vi "checkBeginPassPlay.vi"(8 "error in (no error)":errorcluster, 10 "Game":refnum<class "Game.lvclass">, 11 "PassPlay in":refnum<class "PassPlay.lvclass">) -> (0 "error out":errorcluster, 2 "Boolean":bool, 3 "PassPlay out":refnum<class "PassPlay.lvclass">)   [LabVIEW 2023, in "PassPlay.lvclass"]
uses:
  PassPlay.lvclass
  Game_class/Game.lvclass
  Utilities_class/Utilities.lvclass
  Referee_class/command_interpreted.ctl
  Game_class/Game.lvclass/Game.ctl
  Referee_class/Referee.lvclass/Referee.ctl
  Game_class/Read Referee.vi
  Referee_class/Read command_interpreted.vi
  Referee_class/Referee.lvclass
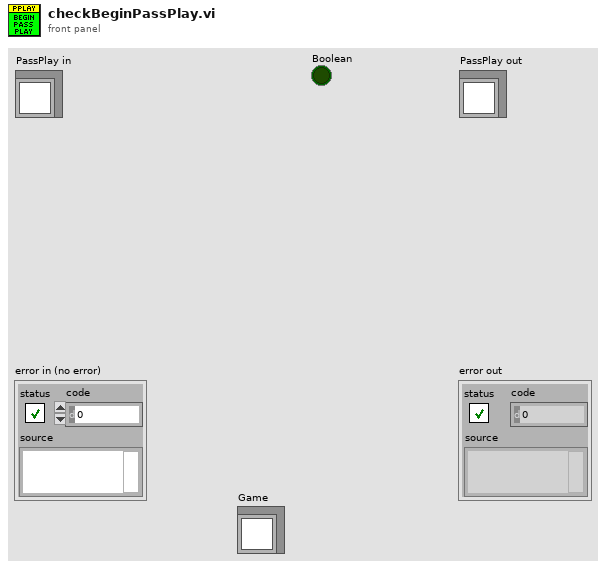
[diagram p1: front panel]
types:
  T1 = typedef "command_interpreted.ctl" = enum16{"Goal Ally", "Goal Enemy", "Ball Placement Enemy", "Ball Placement Ally", "Normal Half Time", "Extra Time  Break", "Extra Half Time", "None", "Post Game", "PKA Normal Start", "Prepare Kickoff Ally", "PKE Normal Start", "Prepare Kickoff Enemy", "Force Start", "Halt", "Timeout", "Prepare Penalty Ally", "Prepare Penalty Enemy", "PPA NormalStart", "PPE Normal Start", "Indirect Free Ally", "Direct Free Enemy", "Direct Free Ally", "Indirect Free Enemy", "Stop"}
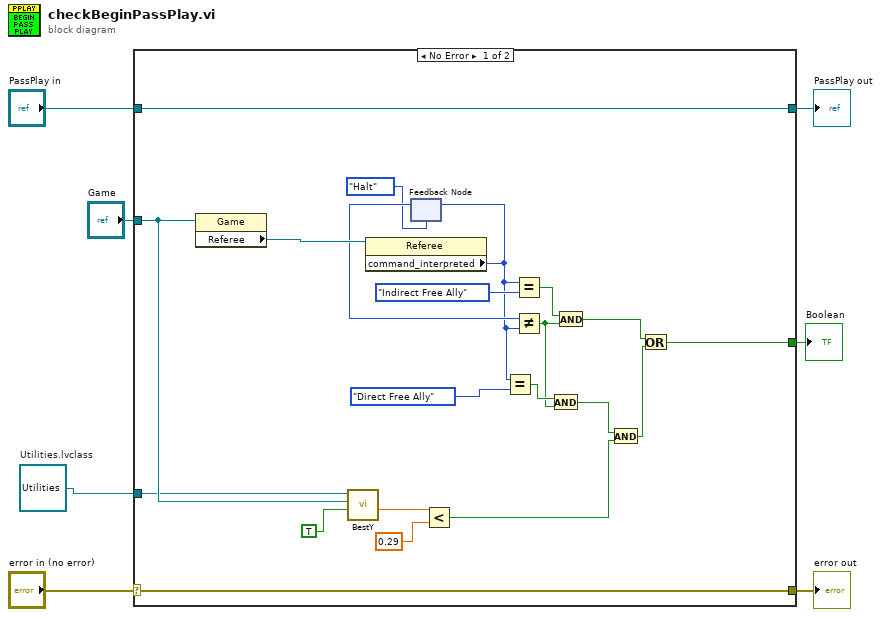
[diagram p0: block diagram]
diagram:
  w1 = refnum<class "Utilities.lvclass"> refnum  # Utilities.lvclass
  n1 = case shown="No Error" "error in (no error)" {
    selector: "error in (no error)" -> [w27 w30]
    tunnel: [w27 w30] -> w6
    tunnel: [w28 w29] -> w4
    tunnel: "PassPlay in" -> [w28 w29]
    tunnel: "Game" -> [w13 _]
    tunnel: [w14 _] -> w2
    tunnel: w1 -> [w9 _]
    frame No Error {
      n2 = property class="Game"(reference=w13) -> ("Referee"=w26:refnum<class "Referee.lvclass">)  [unwired: 1 in, 2 out]
      n3 = call "BestY.vi"("Utilities in"=w9, "Game"=w13, "inimigos"=TRUE) -> ("Gap kick"=w12:dbl)  [unwired: 2 in, 4 out]
      n4 = property class="Referee"(reference=w26) -> ("command_interpreted"=w21:T1)  [unwired: 1 in, 2 out]
      n5 = feedback #1(command_interpreted."Halt" ("command_interpreted")) -> (w23:T1)
      n6 = feedback-in #1(w21) -> ()
      n7 = Less?(x=w12, y=0.29) -> (x < y?=w10:bool)
      n8 = Equal?(x=w21, y=command_interpreted."Direct Free Ally" ("command_interpreted")) -> (x = y?=w19:bool)
      n9 = Equal?(x=w21, y=command_interpreted."Indirect Free Ally" ("command_interpreted")) -> (x = y?=w24:bool)
      n10 = Not Equal?(x=w23, y=w21) -> (x != y?=w18:bool)
      n11 = And(x=w19, y=w18) -> (x .and. y?=w16:bool)
      n12 = And(x=w24, y=w18) -> (x .and. y?=w17:bool)
      n13 = And(x=w16, y=w10) -> (x .and. y?=w15:bool)
      n14 = Or(x=w17, y=w15) -> (x .or. y?=w14:bool)
    }
    frame Error {
    }
  }
  "error out" <- w6
  "PassPlay out" <- w4
  "Boolean" <- w2
